vi "DataLoggerBuildTags.vi"(8 "error in (no error)":errorcluster, 10 "Config":cluster{"Tag List":string[]}, 11 "ModuleID":string) -> (0 "error out":errorcluster, 3 "Tag Refs":T1)   [LabVIEW 2020, in "DataLogger.lvlib"]
uses:
  DataLogger.lvlib
  3621d97f-605c-4e6f-807d-a17beb1ed3ae.vi
  f8fd6500-b03e-4021-a7cb-1885c161f361.vi
  74357129-81d6-44a7-b1a0-f4ce26dbfdd0.vi
  <vilib>/Tag Engine/Tag/Tag.lvclass
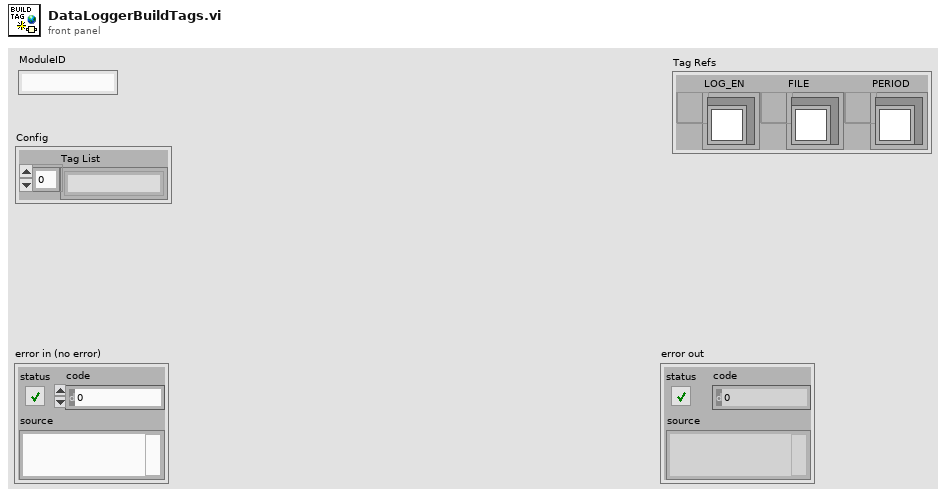
[diagram p1: front panel]
types:
  T1 = cluster{"LOG_EN":refnum<data-value>, "FILE":refnum<data-value>, "PERIOD":refnum<data-value>}
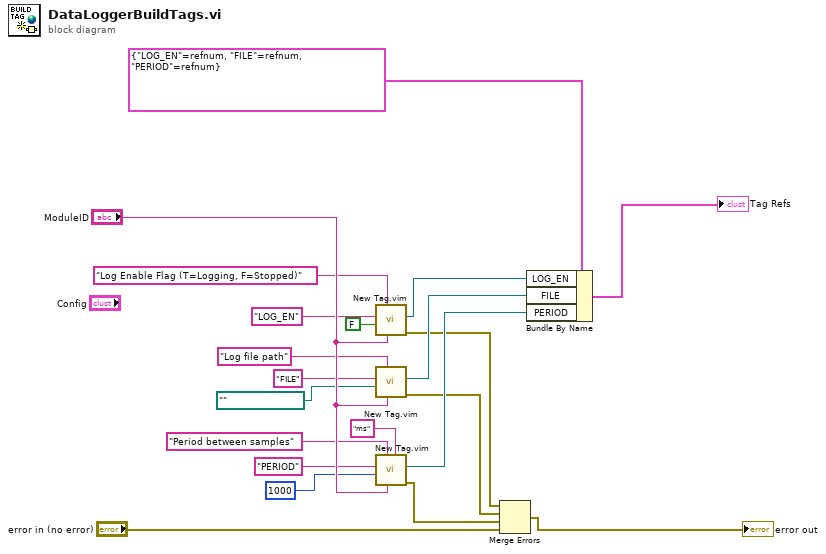
[diagram p0: block diagram]
diagram:
  n1 = call "New Tag.vim"("Namespace"="ModuleID", "Description (none)"="Log Enable Flag (T=Logging, F=Stopped)", "Initial Value"=FALSE, "Tag Name"="LOG_EN") -> ("error out"=w7:errorcluster, "Tag Ref out"=w10:refnum<data-value>)  [unwired: 6 in]
  n2 = call "New Tag.vim"("Namespace"="ModuleID", "Description (none)"="Log file path", "Initial Value"=path "", "Tag Name"="FILE") -> ("error out"=w6:errorcluster, "Tag Ref out"=w9:refnum<data-value>)  [unwired: 6 in]
  n3 = call "New Tag.vim"("Units (none)"="ms", "Namespace"="ModuleID", "Description (none)"="Period between samples", "Initial Value"=1000 ("millisecond multiple"), "Tag Name"="PERIOD") -> ("error out"=w5:errorcluster, "Tag Ref out"=w8:refnum<data-value>)  [unwired: 5 in]
  n4 = Merge Errors(w7, w6, w5, "error in (no error)") -> (→"error out":errorcluster)
  n5 = Bundle By Name(cluster=T1 {"LOG_EN"=refnum, "FILE"=refnum, "PERIOD"=refnum} ("Tag Refs"), "LOG_EN"=w10, "FILE"=w9, "PERIOD"=w8) -> (→"Tag Refs":T1)
